vi "Update Digital Audio Generation (Freq and Amp).vi"(8 "error in (no error)":errorcluster, 9 "gain":dbl, 10 "frequency":dbl, 11 "PCM tasks":T1) -> (0 "error out":errorcluster, 3 "PCM tasks":T1)   [LabVIEW 2021]
uses:
  <vilib>/PDM Acquisition Toolkit/host/Classes/Channels/PCM Output/PCM Output Channel.lvclass
  C:/Program Files/National Instruments/LabVIEW 2021/vi.lib/PDM Acquisition Toolkit/host/Classes/Channels/DecoderChannel.lvclass
  <vilib>/PDM Acquisition Toolkit/host/Classes/Channels/PCM Output/controls/PCM Output Channel - Signal Properties.ctl
  <vilib>/PDM Acquisition Toolkit/host/Classes/Channels/DecoderChannel.lvclass
  <vilib>/PDM Acquisition Toolkit/host/Classes/Tasks/PCM Output/PCM Output Task.lvclass
  C:/Program Files/National Instruments/LabVIEW 2021/vi.lib/PDM Acquisition Toolkit/host/Classes/Channels/PCM Output/PCM Output Channel.lvclass
  <vilib>/PDM Acquisition Toolkit/host/Classes/Tasks/PCM Output/Controls/PCM Output Task DVR.ctl
  controls/digital audio protocol/PCM tasks.ctl
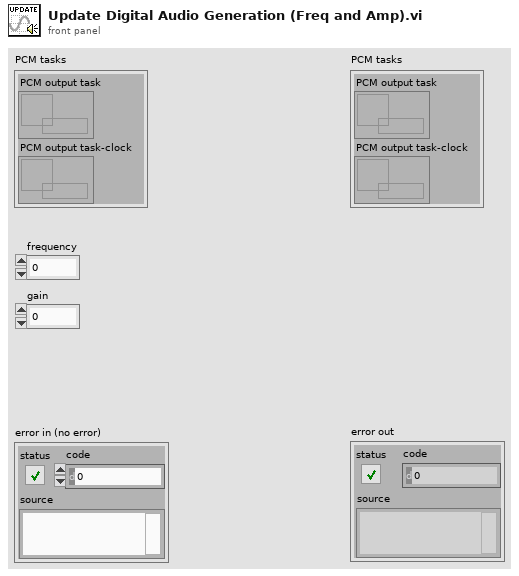
[diagram p1: front panel]
types:
  T1 = typedef "PCM tasks.ctl" = cluster{"PCM output task":T2, "PCM output task-clock":T2}
  T2 = typedef "PDM Acquisition Class Library.lvlib/PCM Output Task.lvclass/PCM Output Task DVR.ctl" = refnum<data-value>
  T3 = typedef "PDM Acquisition Class Library.lvlib/PCM Output Channel.lvclass/PCM Output Channel - Signal Properties.ctl" = cluster{"cyclic period":dbl, "cyclic phase offset":dbl, "gain":dbl}
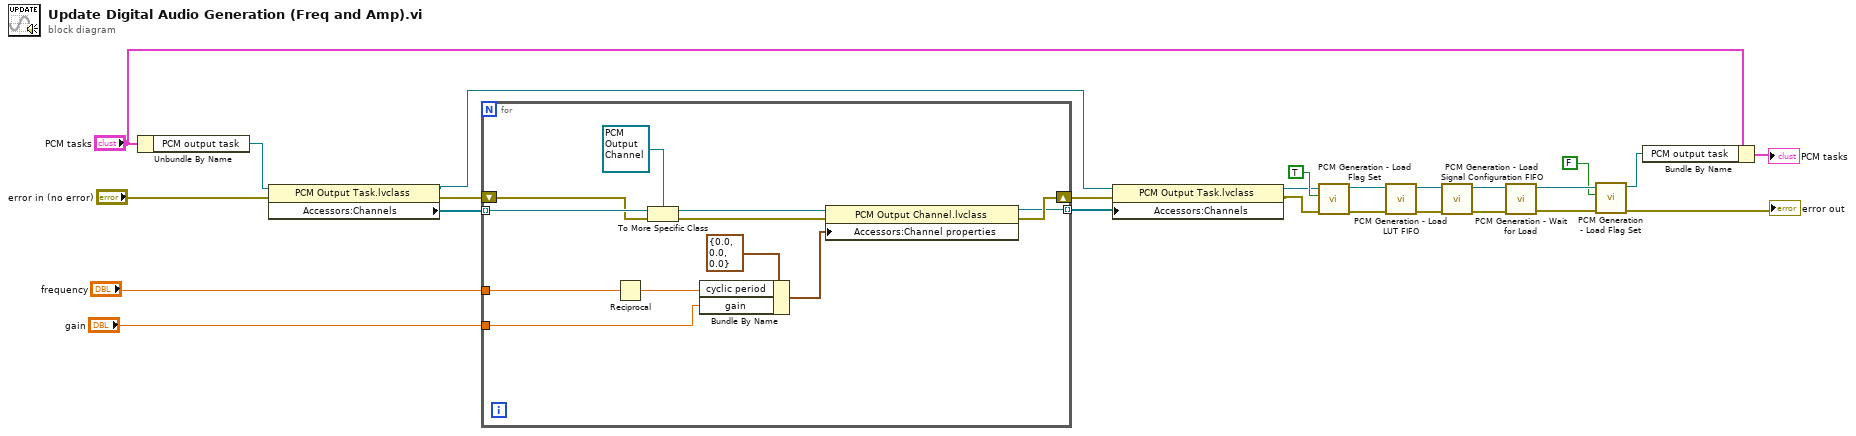
[diagram p0: block diagram]
diagram:
  n1 = Unbundle By Name("PCM tasks") -> ("PCM output task"=w4:T2)
  n2 = property class="PCM Output Task.lvclass"(reference=w4, error in="error in (no error)") -> (reference out=w12:T2, error out=w24:errorcluster, "Accessors:Channels"=w25:refnum<class "DecoderChannel.lvclass">[])
  n3 = for {
    tunnel: w25 -> [w36] mode=indexing
    shift-right: [w32] -> w14
    shift-left: w24 -> [w34]
    tunnel: [w31] -> w13 mode=indexing
    tunnel: "frequency" -> [w27]
    tunnel: "gain" -> [w26]
    n4 = Reciprocal(x=w27) -> (1/x=w30:dbl)
    n5 = To More Specific Class(target class=refnum<class "PCM Output Channel.lvclass"> refnum ("PDM Acquisition Class Library.lvlib:PCM Output Channel.lvclass"), reference=w36, error in=w34) -> (specific class reference=w33:refnum<class "PCM Output Channel.lvclass">, error out=w37:errorcluster)
    n6 = Bundle By Name(cluster=T3 {"cyclic period"=0.0, "cyclic phase offset"=0.0, "gain"=0.0} ("Channel properties"), "cyclic period"=w30, "gain"=w26) -> (w28:T3)
    n7 = property class="PCM Output Channel.lvclass"(reference=w33, error in=w37, "Accessors:Channel properties"=w28) -> (reference out=w31:refnum<class "PCM Output Channel.lvclass">, error out=w32:errorcluster)
  }
  n8 = property class="PCM Output Task.lvclass"(reference=w12, error in=w14, "Accessors:Channels"=w13) -> (reference out=w11:T2, error out=w10:errorcluster)
  n9 = call <vilib>:"PCM Generation - Load Flag Set.vi"("error in"=w10, "Load"=TRUE, "PCM Output Task In"=w11) -> ("error out"=w18:errorcluster, "PCM Output Task Out"=w17:T2)  [unwired: 7 in]
  n10 = call <vilib>:"PCM Generation - Load LUT FIFO.vi"("error in"=w18, "PCM Output Task In"=w17) -> ("error out"=w15:errorcluster, "PCM Output Task Out"=w16:T2)  [unwired: 8 in]
  n11 = call <vilib>:"PCM Generation - Load Signal Configuration FIFO.vi"("error in"=w15, "PCM Output Task In"=w16) -> ("error out"=w9:errorcluster, "PCM Output Task Out"=w19:T2)  [unwired: 8 in]
  n12 = call <vilib>:"PCM Generation - Wait for Load.vi"("error in"=w9, "PCM Output Task In"=w19) -> ("error out"=w21:errorcluster, "PCM Output Task Out"=w22:T2)  [unwired: 7 in, 1 out]
  n13 = call <vilib>:"PCM Generation - Load Flag Set.vi"("error in"=w21, "Load"=FALSE, "PCM Output Task In"=w22) -> ("error out"=→"error out":errorcluster, "PCM Output Task Out"=w1:T2)  [unwired: 7 in]
  n14 = Bundle By Name(cluster="PCM tasks", "PCM output task"=w1) -> (→"PCM tasks":T1)
